vi "SerialViewer.vi"() -> ()   [LabVIEW 2018, in "Serial.lvlib"]
uses:
  Serial.lvlib
  <vilib>/Platform/TimedLoop/XDataNode/timing_clust.ctl
  <vilib>/Platform/TimedLoop/XDataNode/nitl_modes.ctl
  <vilib>/Platform/TimedLoop/XDataNode/wakeup.ctl
  <vilib>/Instr/_visa.llb/VISA Configure Serial Port (Instr).vi
  <vilib>/platform/TimedLoop/XDataNode/XDataNode.xnode
  <vilib>/Platform/TimedLoop/XDataNode/XDNodeRunTimeDep.lvlib
panel:
  out "Values #3":dbl(graph)
  in  "?":enum32{"Reading", "Communication", "Loop"}(tab)
  out "Value #2":dbl
  out "Value #1":dbl
  in  "Count":u32=1000
  out "Data 1D":dbl[](array[numeric]) caption="array" format="%#_2f"
  in  "Process input":bool
  in  "Baud":enum16{"9600", "19200", "57600", "115200"}(ring)
  in  "Serial port":refnum<visa-resource-name>="COM1"
  in  "Frequency":dbl(slide) scale=1.0..100.0
  in  "Stop":bool
  out "Counter":i32
  out "Interval":i64
  out "Values #1":dbl(graph)=-207.0
  out "Values #2":dbl(graph)
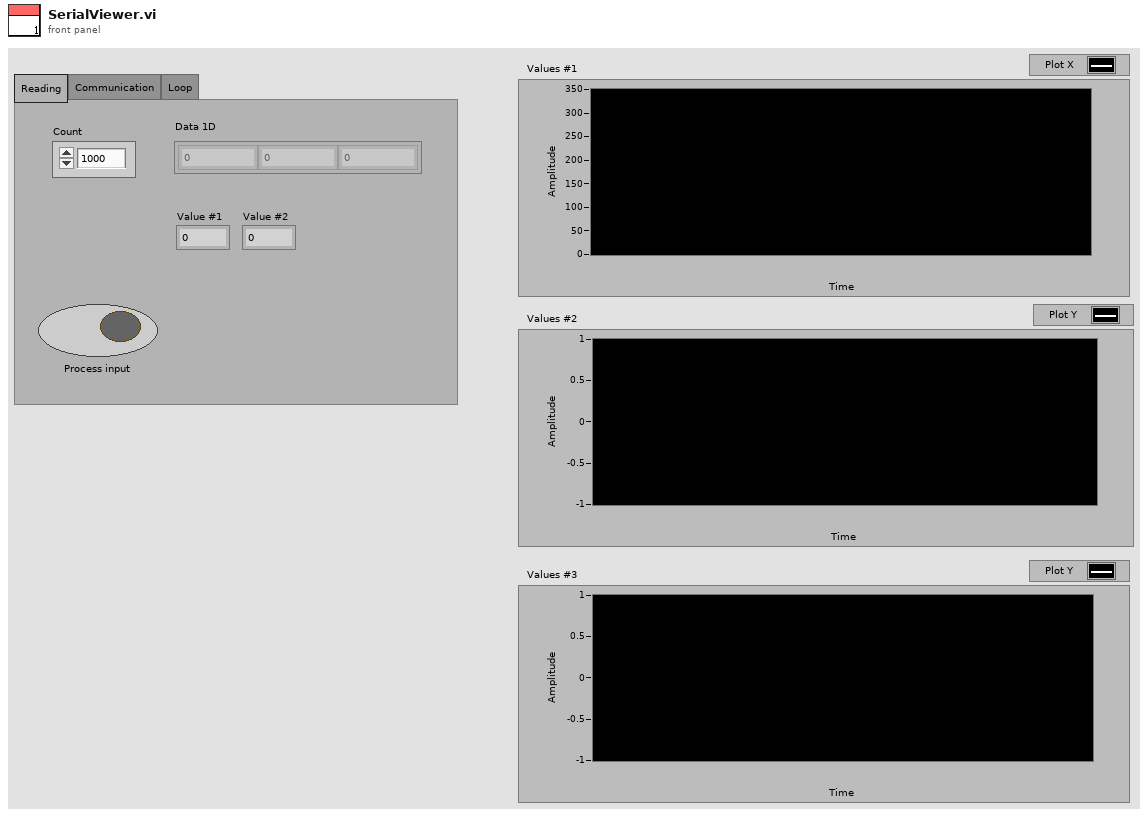
[diagram p1: front panel]
types:
  T1 = typedef "XDNodeRunTimeDep.lvlib/timing_clust.ctl" = cluster{"Expected End [f-1]":u64, "Actual End [f-1]":u64, "Finished Late? [f-1]":bool, "Expected End [i-1]":u64, "Actual End [i-1]":u64, "Finished Late? [i-1]":bool, "Expected Start [i]":u64, "Actual Start [i]":u64, "Expected Start [f]":u64, "Actual Start [f]":u64, "Source Name":string, "Structure Name":string, "Period":i64, "Deadline":i64, "Offset":i64, "Start":i64, "Priority":i32, "Timeout":i32, "Mode":T2, "Wakeup Reason":T3, "Error":errorcluster, "Source Type":string, "Secondary Source Type":string, "Global End Time":u64, "Global Start Time":u64, "Frame Duration":u64, "Iteration Duration":u64, "Assigned CPU":i32, "I/O Scan Engine Mode":u32}
  T2 = typedef "XDNodeRunTimeDep.lvlib/nitl_modes.ctl" = enum32{"No Change", "Process missed periods, maintain original phase", "Discard missed periods, maintain original phase", "Process missed periods, ignore original phase", "Discard missed periods, ignore original phase"}
  T3 = typedef "XDNodeRunTimeDep.lvlib/wakeup.ctl" = enum32{"Normal", "Aborted", "Asynchronous wakeup", "Timing source error", "Timed loop error", "Timeout"}
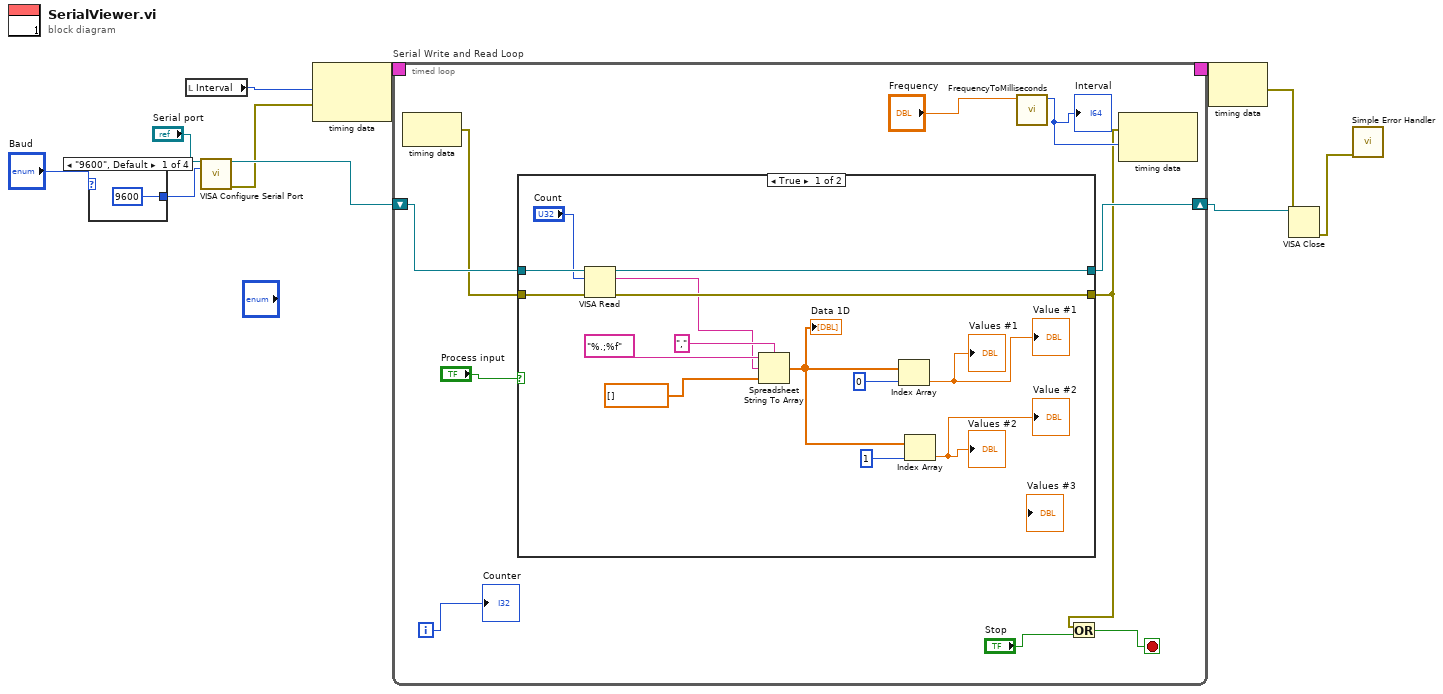
[diagram p0: block diagram]
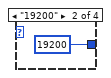
[diagram p2: hidden frame]
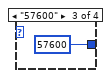
[diagram p3: hidden frame]
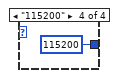
[diagram p4: hidden frame]
diagram:
  n1 = case shown="\"9600\", Default" "Baud" {
    tunnel: [u32 9600 ("baud rate (9600)") u32 19200 ("baud rate (9600)") u32 57600 ("baud rate (9600)") u32 115200 ("baud rate (9600)")] -> w1
    frame "9600", Default {
    }
    frame "19200" {
    }
    frame "57600" {
    }
    frame "115200" {
    }
  }
  n2 = local read "Interval"() -> (w9:i64)
  n3 = call-poly "VISA Configure Serial Port"("VISA resource name"="Serial port", "baud rate (9600)"=w1) -> ("VISA resource name out"=w8:refnum<visa-resource-name>, "error out"=w7:errorcluster)  [unwired: 8 in, 4 out]
  n4 = node-c288(w9, w7) -> (w11:T1)
  n5 = timed-loop "Serial Write and Read Loop" {
    timing: w11 -> [_]
    timing-out: [_] -> w10
    shift-right: [w18] -> w4
    shift-left: w8 -> [w20]
    i -> [w23]
    stop <- w22 stop-if-true
    n6 = node-c288() -> (w19:errorcluster)  [unwired: 1 in]
    n7 = case shown="True" "Process input" {
      tunnel: [w37 w41] -> w18
      tunnel: w20 -> [w39 w41]
      tunnel: [w35 w40] -> w16
      tunnel: w19 -> [w38 w40]
      frame True {
        n8 = VISA Read(VISA resource name=w39, byte count="Count", error in (no error)=w38) -> (VISA resource name out=w37:refnum<visa-resource-name>, read buffer=w31:string, error out=w35:errorcluster)  [unwired: 1 out]
        n9 = Spreadsheet String To Array(delimiter (Tab)=",", format string="%.;%f", spreadsheet string=w31, array type (2D Dbl)=dbl[] [] ("Data Graph")) -> (array=w28:dbl[])
        "Data 1D" <- w28
        n10 = Index Array(array=w28, index=0 ("disabled index (col)")) -> (element=→"Values #1" →"Value #1":dbl)
        n11 = Index Array(array=w28, index=1 ("disabled index (col)")) -> (element=→"Values #2" →"Value #2":dbl)
      }
      frame False {
      }
    }
    n12 = call "FrequencyToMilliseconds.vi"("Frequency"="Frequency") -> ("Numeric"=w24:i64)  [unwired: 10 in]
    "Interval" <- w24
    n13 = Or(x=w16, y="Stop") -> (x .or. y?=w22:bool)
    n14 = node-c288(w16, w24) -> ()  [unwired: 1 out]
    "Counter" <- w23
  }
  n15 = node-c288(w10) -> (w5:errorcluster)
  n16 = VISA Close(VISA resource name=w4, error in (no error)=w5) -> (error out=w3:errorcluster)
  n17 = call <vilib>:"Simple Error Handler.vi"("error in (no error)"=w3) -> ()  [unwired: 1 in, 8 out]
